vi "VeriStand Framework.Create.vi"(8 "error in (no error)":errorcluster, 10 "Engine Data Ref":T1 {"Ptr.End" format="%.0x"; "Ptr.Beg" format="%.0x"}, 11 "Device Item Ref":T2=18446744073709551615 format="%.0x") -> (0 "error out":errorcluster, 3 "VeriStand Framework out":refnum<class "VeriStand Framework.lvclass">)   [LabVIEW 2017, in "Data Sharing Framework Engine.lvlib" / "VeriStand Framework.lvclass"]
uses:
  VeriStand Framework.lvclass
  <vilib>/NI Veristand/Custom Device API/Custom Device Item Ref.ctl
  <vilib>/NI Veristand/Custom Device API/Data Table Ref.ctl
  DSF Core/Built/Windows/Engine/DSF.Engine.lvlibp/Engine/Classes/Pointer/DSF.Engine.Pointer.DBL.lvclass
  VeriStand Framework.lvclass/VeriStand Framework.ctl
  DSF Core/Built/Windows/Dependencies/Memory Manager.lvlibp/1abvi3w/vi.lib/National Instruments/Memory Manager/Classes/Pointer/Memory.Pointer.lvclass
  DSF Core/Built/Windows/Engine/DSF.Engine.lvlibp/Engine/Classes/Framework/DSF.Engine.Framework.lvclass
  C:/Git/DSF/DSF Core/Built/Windows/Dependencies/Memory Manager.lvlibp/1abvi3w/vi.lib/National Instruments/Memory Manager/Classes/Pointer/Memory.Pointer.lvclass
  C:/Git/DSF/DSF Core/Built/Windows/Engine/DSF.Engine.lvlibp/Engine/Classes/Framework/DSF.Engine.Framework.lvclass
  <vilib>/NI Veristand/Custom Device API/Custom Device API.lvlib
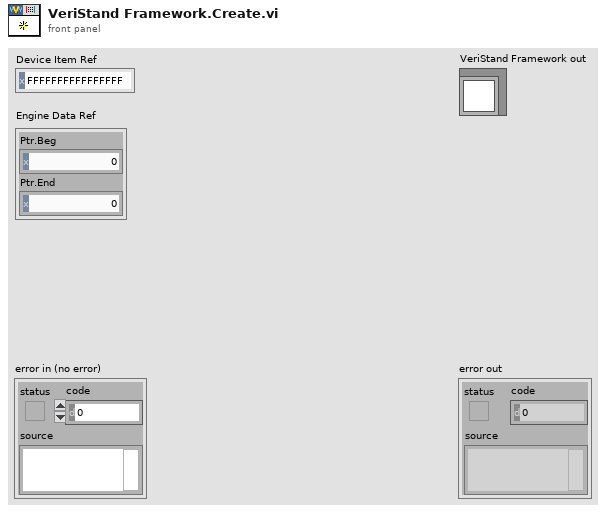
[diagram p1: front panel]
types:
  T1 = typedef "Custom Device API.lvlib/Data Table Ref.ctl" = cluster{"Ptr.Beg":u64, "Ptr.End":u64}
  T2 = typedef "Custom Device API.lvlib/Custom Device Item Ref.ctl" = u64
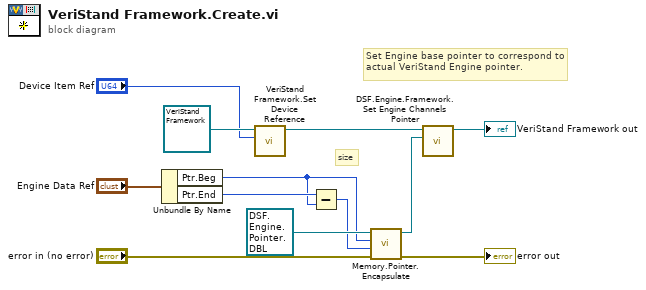
[diagram p0: block diagram]
diagram:
  # "size"
  # "Set Engine base pointer to correspond to actual VeriStand Engine pointer."
  n1 = Unbundle By Name("Engine Data Ref") -> ("Ptr.Beg"=w2:u64, "Ptr.End"=w4:u64)
  n2 = call "VeriStand Framework.Set Device Reference.vi"("Device Item Ref"="Device Item Ref", "VeriStand Framework in"=refnum<class "VeriStand Framework.lvclass"> refnum) -> ("VeriStand Framework out"=w6:refnum<class "VeriStand Framework.lvclass">)  [unwired: 9 in]
  n3 = Subtract(x=w4, y=w2) -> (x-y=w3:u64)
  n4 = call "Memory.Pointer.Encapsulate.vi"("error in (no error)"="error in (no error)", "size"=w3, "address"=w2, "Pointer type"=refnum<class "DSF.Engine.Pointer.DBL.lvclass"> refnum ("Engine Channels Pointer")) -> ("error out"=→"error out":errorcluster, "Pointer out"=w1:refnum<class "DSF.Engine.Pointer.DBL.lvclass">)  [unwired: 6 in]
  n5 = call "DSF.Engine.Framework.Set Engine Channels Pointer.vi"("Engine Channels Pointer"=w1, "Framework in"=w6) -> ("Framework out"=→"VeriStand Framework out":refnum<class "VeriStand Framework.lvclass">)  [unwired: 9 in]
